vi "Utility Log to File.vi"(8 "error in (no error)":errorcluster, 10 "Command":string, 11 "Log File Path":path) -> (0 "error out":errorcluster)   [LabVIEW 2020, in "Omega Platinum Series.lvlib"]
doc: "Logs a given command to the specified logging file. A timestamp of the current time is logged with the command, along with any error codes present in the \"error in\" parameter. The \"error out\" return value only returns errors from the logging itself; errors present in the \"error in\" parameter are ignored and used for logging purposes only."
uses:
  Omega Platinum Series.lvlib
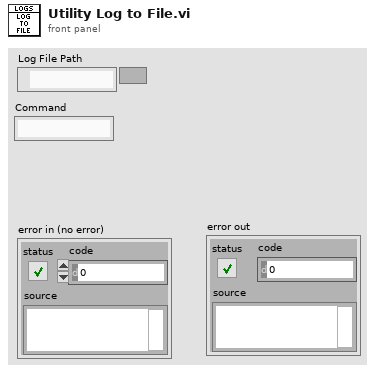
[diagram p1: front panel]
types:
  T1 = enum16{"open", "replace", "create", "open or create", "replace or create", "replace or create with confirmation"}
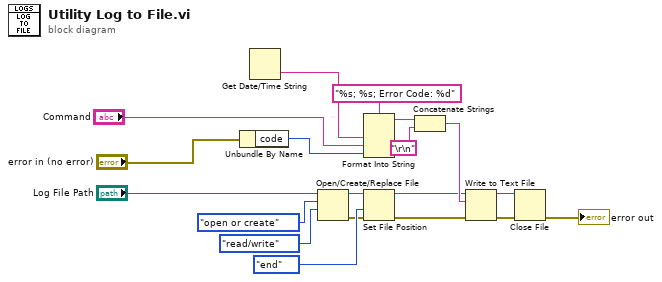
[diagram p0: block diagram]
diagram:
  n1 = Unbundle By Name("error in (no error)") -> ("code"=w16:i32)
  n2 = Get Date/Time String() -> (time string=w17:string)  [unwired: 3 in, 1 out]
  n3 = Open/Create/Replace File(file path (use dialog)="Log File Path", operation (0:open)=T1."open or create", access (0:read/write)=enum16{"read/write", "read-only", "write-only"}."read/write") -> (refnum out=w4:refnum<file>, error out=w3:errorcluster)  [unwired: 3 in, 1 out]
  n4 = Format Into String(format string="%s; %s; Error Code: %d", w17, "Command", w16) -> (resulting string=w13:string)  [unwired: 2 in, 1 out]
  n5 = Set File Position(refnum=w4, from (0:start)=enum16{"start", "end", "current"}."end", error in=w3) -> (refnum out=w6:refnum<file>, error out=w5:errorcluster)  [unwired: 1 in]
  n6 = Concatenate Strings(w13, "\r\n") -> (w14:string)
  n7 = Write to Text File(file (use dialog)=w6, text=w14, error in=w5) -> (refnum out=w8:refnum<file>, error out=w7:errorcluster)  [unwired: 1 in, 1 out]
  n8 = Close File(refnum=w8, error in=w7) -> (error out=→"error out":errorcluster)  [unwired: 1 out]
